vi "Apply Individual Gradient.vi"(8 "error in":errorcluster, 9 "Current [A]":dbl format="%.3f", 10 "Gradient Supply Address":string, 11 "Gradient Supply Type":string) -> (0 "error out":errorcluster)   [LabVIEW 2016]
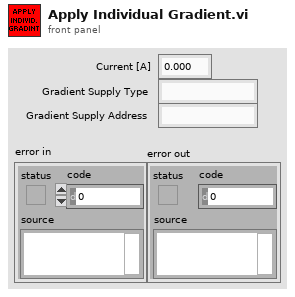
[diagram p1: front panel]
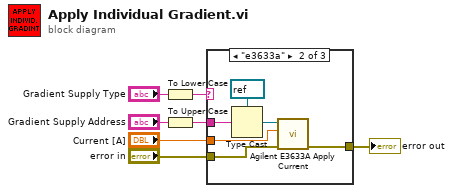
[diagram p0: block diagram]
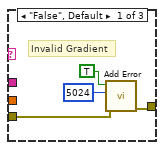
[diagram p2: hidden frame]
diagram:
  n1 = To Lower Case(string="Gradient Supply Type") -> (all lower case string=w6:string)
  n2 = To Upper Case(1:"Gradient Supply Address") -> (0:w3:string)
  n3 = case shown="\"e3633a\"" w6 {
    tunnel: [w10 w14 w18] -> w2
    tunnel: "error in" -> [w11 w15 w18]
    tunnel: w3 -> [_ w17 _]
    tunnel: "Current [A]" -> [_ w12 _]
    frame "False", Default {
      # "Invalid Gradient"
      n4 = call "Add Error.vi"("error in (no error)"=w11, "error code (0)"=5024, "error?"=TRUE) -> ("error out"=w10:errorcluster)  [unwired: 8 in]
    }
    frame "e3633a" {
      n5 = Type Cast(type=refnum<k15> refnum ("resource name"), x=w17) -> (*(type *) &x=w13:refnum<k15>)
      n6 = call "Agilent E3633A Apply Current.vi"("error in (no error)"=w15, "Current [A]"=w12, "resource name"=w13) -> ("error out"=w14:errorcluster)  [unwired: 5 in, 1 out]
    }
    frame "rri_loadgo" {
    }
  }
  "error out" <- w2
